vi "HEWH Index Start of Draw By Program Status.vi"(9 "Elapsed Time (sec)":dbl, 10 "Data Type":T1, 11 "Program Status":string) -> (2 "Purging":i16, 3 "Drawing":i16)   [LabVIEW 2023]
uses:
  Type Definitions/HEWH Meter Type.ctl
  <vilib>/Utility/error.llb/whitespace.ctl
  <vilib>/Utility/error.llb/Trim Whitespace One-Sided.vi
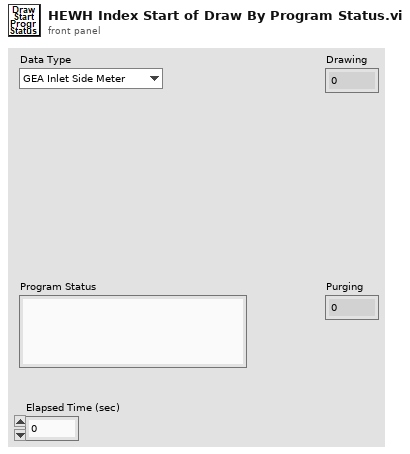
[diagram p1: front panel]
types:
  T1 = typedef "HEWH Meter Type.ctl" = enum16{"GEA Inlet Side Meter", "GEA Outlet Side Meter", "CSA Inlet Side Meter"}
  T2 = typedef "whitespace.ctl" = u16
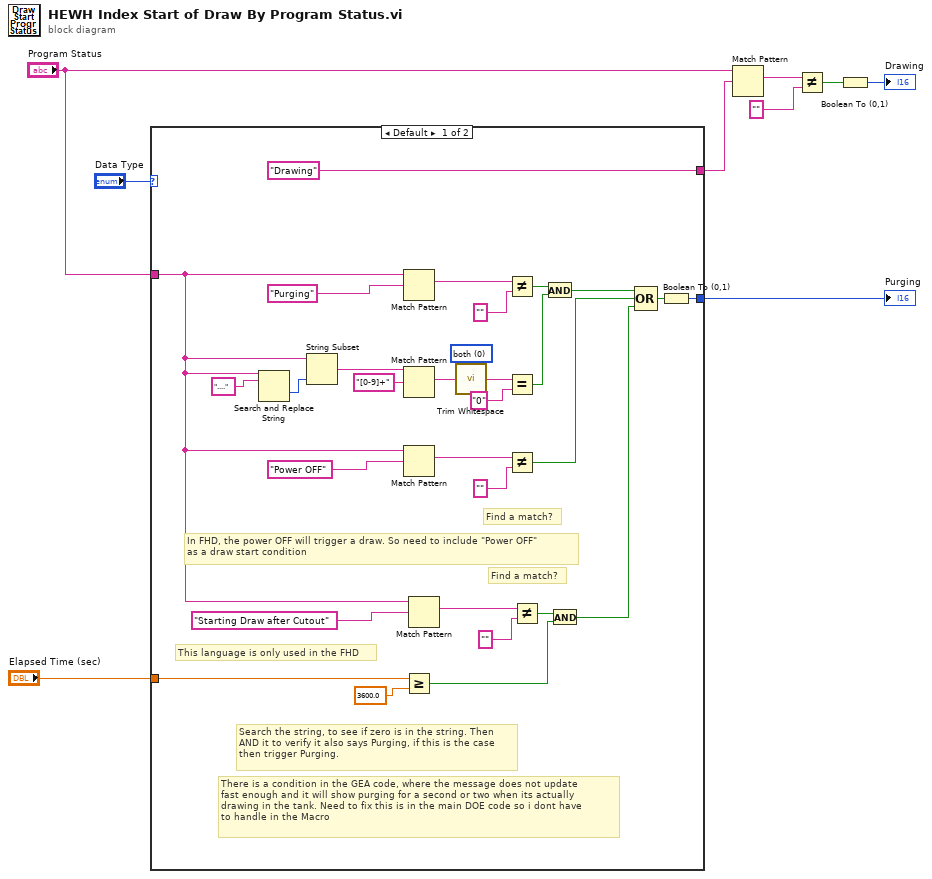
[diagram p0: block diagram]
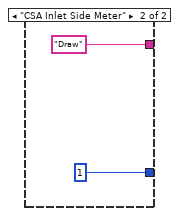
[diagram p2: hidden frame]
diagram:
  n1 = case shown="Default" "Data Type" {
    tunnel: ["Drawing" ("regular expression") "Draw" ("regular expression")] -> w6
    tunnel: [w25 i16 1 ("0, 1")] -> w2
    tunnel: "Program Status" -> [w15 _]
    tunnel: "Elapsed Time (sec)" -> [w13 _]
    frame Default {
      w30 = T2 0 items=["both", "start of string", "end of string"] ("location (both)")
      # "Find a match?"
      # "Find a match?"
      # "This language is only used in the FHD"
      # "In FHD, the power OFF will trigger a draw. So need to include \"Power OFF\"\nas a draw start condition"
      # "There is a condition in the GEA code, where the message does not update\nfast enough and it will show purging for a second or two when its actually \ndrawing in the tank. Need to fix this is in the main DOE code so i dont have \nto handle in the Macro"
      # "Search the string, to see if zero is in the string. Then\nAND it to verify it also says Purging, if this is the case\nthen trigger Purging."
      n2 = Search and Replace String(input string=w15, search string="....") -> (offset past replacement=w33:i32)  [unwired: 6 in, 3 out]
      n3 = String Subset(string=w15, length (rest)=w33) -> (substring=w34:string)  [unwired: 1 in]
      n4 = Match Pattern(string=w15, regular expression="Purging") -> (match substring=w32:string)  [unwired: 1 in, 3 out]
      n5 = Match Pattern(string=w34, regular expression="[0-9]+") -> (match substring=w35:string)  [unwired: 1 in, 3 out]
      n6 = Match Pattern(string=w15, regular expression="Power OFF") -> (match substring=w22:string)  [unwired: 1 in, 3 out]
      n7 = Greater Or Equal?(x=w13, y=3600.0) -> (x >= y?=w11:bool)
      n8 = Match Pattern(string=w15, regular expression="Starting Draw after Cutout") -> (match substring=w18:string)  [unwired: 1 in, 3 out]
      n9 = call <vilib>:"Trim Whitespace.vi"("string"=w35, "location (both)"=w30) -> ("trimmed string"=w36:string)
      n10 = Not Equal?(x=w32, y="") -> (x != y?=w38:bool)
      n11 = Equal?(x=w36, y="0") -> (x = y?=w37:bool)
      n12 = Not Equal?(x=w22, y="") -> (x != y?=w20:bool)
      n13 = Not Equal?(x=w18, y="") -> (x != y?=w14:bool)
      n14 = And(x=w38, y=w37) -> (x .and. y?=w21:bool)
      n15 = And(x=w14, y=w11) -> (x .and. y?=w10:bool)
      n16 = Compound Arithmetic op=OR(w21, w20, w10) -> (w19:bool)
      n17 = Boolean To (0,1)(Boolean=w19) -> (0, 1=w25:i16)
    }
    frame "CSA Inlet Side Meter" {
    }
  }
  "Purging" <- w2
  n18 = Match Pattern(string="Program Status", regular expression=w6) -> (match substring=w8:string)  [unwired: 1 in, 3 out]
  n19 = Not Equal?(x=w8, y="") -> (x != y?=w9:bool)
  n20 = Boolean To (0,1)(Boolean=w9) -> (0, 1=→"Drawing":i16)
